vi "DrawString.vi"(4 "SpaceTilecode(206)":u32=206, 6 "ColorToReplace (7=white)":fxp<+,3,3>=7.0, 7 "Color (7=white)":fxp<+,3,3>=7.0, 8 "error in (no error)":errorcluster, 9 "Coordinate":T1, 10 "String":string) -> (0 "error out":errorcluster)   [LabVIEW 2019, in "RT_Game.lvlib" / "Engine.lvclass"]
uses:
  Engine.lvclass
  Coordinate.ctl
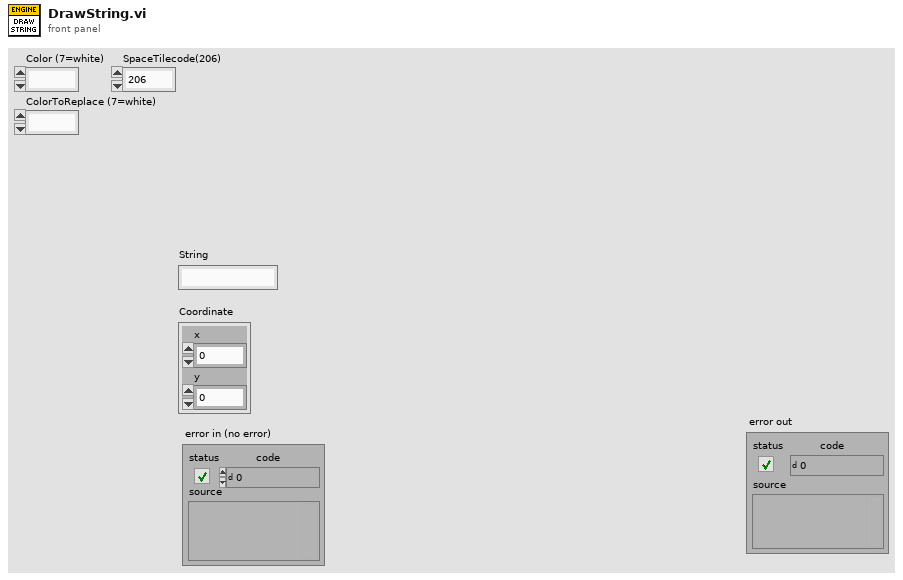
[diagram p1: front panel]
types:
  T1 = typedef "RT_Game.lvlib/Engine.lvclass/Coordinate.ctl" = cluster{"x":dbl, "y":dbl}
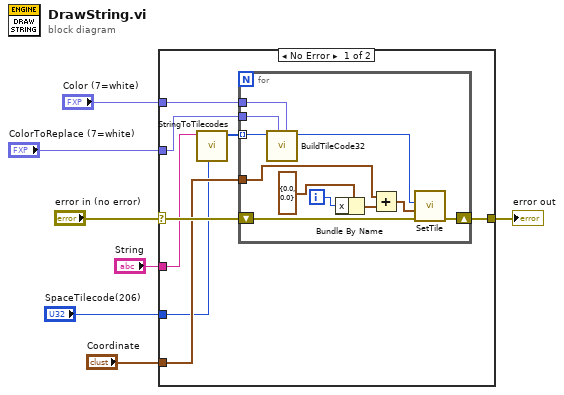
[diagram p0: block diagram]
diagram:
  n1 = case shown="No Error" "error in (no error)" {
    selector: "error in (no error)" -> [w15 w27]
    tunnel: [w14 w27] -> w6
    tunnel: "Coordinate" -> [w13 _]
    tunnel: "String" -> [w9 _]
    tunnel: "Color (7=white)" -> [w12 _]
    tunnel: "ColorToReplace (7=white)" -> [w11 _]
    tunnel: "SpaceTilecode(206)" -> [w8 _]
    frame No Error {
      n2 = call "StringToTilecodes.vi"("SpaceTilecode(206)"=w8, "String"=w9) -> ("Tilecodes"=w10:u32[])  [unwired: 9 in]
      n3 = for {
        shift-right: [w25] -> w14
        shift-left: w15 -> [w26]
        tunnel: w13 -> [w24]
        tunnel: w12 -> [w19]
        tunnel: w11 -> [w18]
        tunnel: w10 -> [w17] mode=indexing
        i -> [w20]
        n4 = call "BuildTileCode32.vi"("replacecolor"=w19, "color_to_replace"=w18, "Tilenumber"=w17) -> ("TileCode"=w16:u32)  [unwired: 8 in]
        n5 = Bundle By Name(cluster=T1 {"x"=0.0, "y"=0.0} ("y"), "x"=w20) -> (w21:T1)
        n6 = Add(x=w24, y=w21) -> (x+y=w23:T1)
        n7 = call "SetTile.vi"("error in (no error)"=w26, "Coordinates"=w23, "TileCode"=w16) -> ("error out"=w25:errorcluster)  [unwired: 8 in]
      }
    }
    frame Error {
    }
  }
  "error out" <- w6
